vi "getNumberOfWheels.vi"(8 "error in (no error)":errorcluster, 11 "genericVehicle in":refnum<class "genericVehicle.lvclass">) -> (0 "error out":errorcluster, 2 "numberOfWheels":dbl, 3 "genericVehicle out":refnum<class "genericVehicle.lvclass">)   [LabVIEW 2011, in "genericVehicle.lvclass"]
uses:
  genericVehicle.lvclass
  genericVehicle.lvclass/genericVehicle.ctl
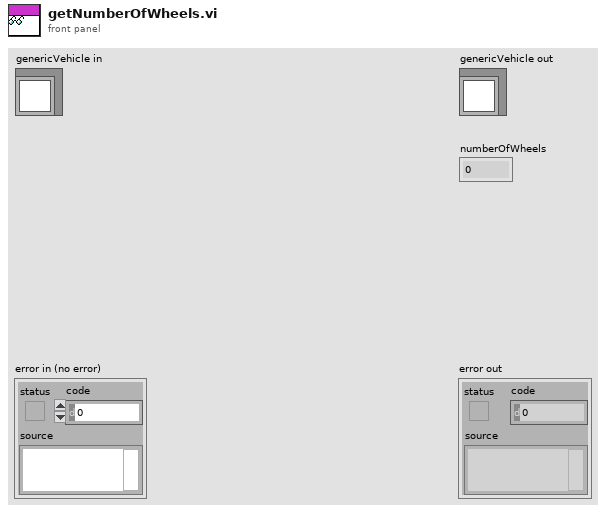
[diagram p1: front panel]
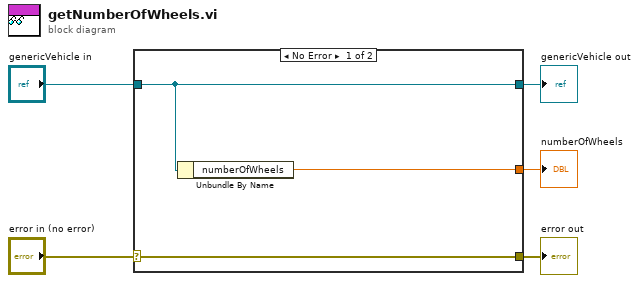
[diagram p0: block diagram]
diagram:
  n1 = case shown="No Error" "error in (no error)" {
    selector: "error in (no error)" -> [w8 w9]
    tunnel: [w8 w9] -> w4
    tunnel: [w7 w10] -> w2
    tunnel: "genericVehicle in" -> [w7 w10]
    tunnel: [w6 _] -> w1
    frame No Error {
      n2 = Unbundle By Name(w7) -> ("numberOfWheels"=w6:dbl)
    }
    frame Error {
    }
  }
  "error out" <- w4
  "genericVehicle out" <- w2
  "numberOfWheels" <- w1
